vi "PCO_SetRecordStopEvent.vi"(8 "error in (no error)":errorcluster {"code" format="%x"}, 9 "dwRecordStopDelayImages":u32, 10 "wRecordStopEventMode":u16(ring) items=["OFF", "software", "extern"], 11 "ph":u64) -> (0 "error out":errorcluster {"code" format="%x"}, 2 "ErrorMessage":i32 format="%x", 3 "ph out":u64)   [LabVIEW 2019, in "SDK.lvlib" / "RecordingControl.lvlib"]
doc: "<b>Description:</b>\nThis function does set the record stop event mode and as an additional parameter the number of images, which will be recorded after a recorder stop event is triggered.\nThe record stop event mode is useful to record a series of images with the ability to review the scene before and after the stop event.\nA record stop event can be triggered through the software command PCO_StopRecord or a signal at the <acq enbl> input. After the stop event is triggered the camera records the configured number of images and stops after that. The record stop event function can only be used if storage mode is set to [recorder] and recorder submode is set to [ring buffer].\nDue to internal timing constrains the current number of images taken after the event may differ by +/- 1 from the configured number.\n\n<b>Supported camera type:</b>\npco.1200, pco.dimax\n\n<b>Descriptor dependency:</b>\ndwGeneralCapsDESC1: RECORD_STOP"
uses:
  RecordingControl.lvlib
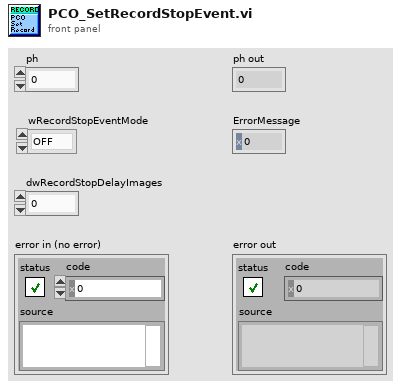
[diagram p1: front panel]
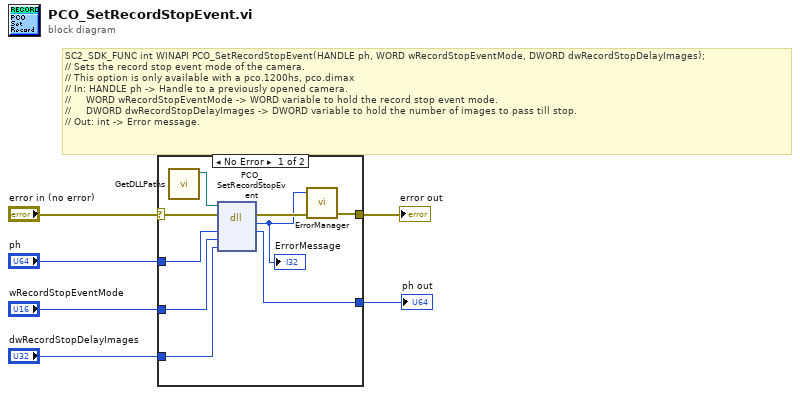
[diagram p0: block diagram]
diagram:
  # "SC2_SDK_FUNC int WINAPI PCO_SetRecordStopEvent(HANDLE ph, WORD wRecordStopEventMode, DWORD dwRecordStopDelayImages);\n// Sets the record stop event mode of the camera.\n// This option is only available with a pco.1200hs, pco.dimax\n// In: HANDLE ph -> Handle to a previously opened camera.\n//     WORD wRecordStopEventMode -> WORD variable to hold the record stop event mode.\n//     DWORD dwRecordStopDelayImages -> DWORD variable to hold the number of images to pass till stop.\n// Out: int -> Error message."
  n1 = case shown="No Error" "error in (no error)" {
    selector: "error in (no error)" -> [w11 w17]
    tunnel: "ph" -> [w15 w16]
    tunnel: [w14 w16] -> w5
    tunnel: "wRecordStopEventMode" -> [w13 _]
    tunnel: "dwRecordStopDelayImages" -> [w12 _]
    tunnel: [w9 w17] -> w2
    frame No Error {
      n2 = call "GetDLLPaths.vi"() -> ("SC2_Cam_Path"=w7:path)  [unwired: 9 in, 2 out]
      n3 = dll-call lib="?" fn="PCO_SetRecordStopEvent"(path in=w7, error in=w11, "ph"=w15, "wRecordStopEventMode"=w13, "dwRecordStopDelayImages"=w12) -> (error out=w10:errorcluster, "return type"=w8:i32, "ph"=w14:u64)  [unwired: 3 in, 1 out]
      "ErrorMessage" <- w8
      n4 = call "ErrorManager.vi"("error in (no error)"=w10, "error code"=w8) -> ("error out"=w9:errorcluster)  [unwired: 3 in]
    }
    frame Error {
    }
  }
  "ph out" <- w5
  "error out" <- w2
